vi "Goomba Movement.vi"(3 "Right Bound":i32=775, 4 "Left Bound":i32=400, 5 "Dir Init":T1, 6 "Pos Init":i32) -> (0 "Picture Name":string, 1 "Dir Out":T1, 2 "Pos Out":i32)   [LabVIEW 2014]
uses:
  Goomba Direction.ctl
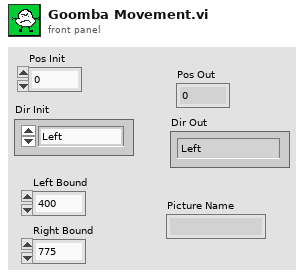
[diagram p1: front panel]
types:
  T1 = typedef "Goomba Direction.ctl" = enum16{"Left", "Right"}
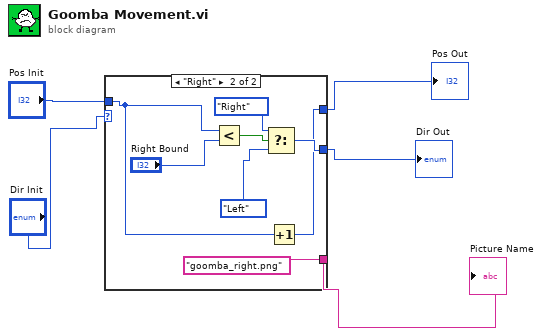
[diagram p0: block diagram]
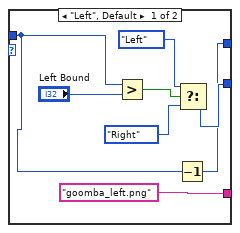
[diagram p2: hidden frame]
diagram:
  n1 = case shown="\"Right\"" "Dir Init" {
    tunnel: [w6 w16] -> w2
    tunnel: "Pos Init" -> [w12 w15]
    tunnel: [w11 w21] -> w3
    tunnel: ["goomba_left.png" "goomba_right.png"] -> w5
    frame "Left", Default {
      n2 = Greater?(x=w12, y="Left Bound") -> (0:w10:bool)
      n3 = Decrement(x=w12) -> (x-1=w6:i32)
      n4 = Select(t=Goomba_Direction."Left", s=w10, f=Goomba_Direction."Right") -> (s? t:f=w11:T1)
    }
    frame "Right" {
      n5 = Less?(x=w15, y="Right Bound") -> (x < y?=w20:bool)
      n6 = Select(t=Goomba_Direction."Right", s=w20, f=Goomba_Direction."Left") -> (s? t:f=w21:T1)
      n7 = Increment(x=w15) -> (x+1=w16:i32)
    }
  }
  "Picture Name" <- w5
  "Dir Out" <- w3
  "Pos Out" <- w2
